vi "NGTS_DAQmx_Initialize_AI.vi"(7 "Save Virtual Channels":bool, 8 "error in":errorcluster, 10 "Channels Properties Table":string[][](array[string])) -> (0 "error out":errorcluster, 2 "AI Task Array Out":refnum<k21>[](array[refnum]))   [LabVIEW 2012]
doc: "Creates tasks based on \"Number_of_SCXI_Chassis\" entry in the AI_Configuration section of the Config_INI file. It then populates the tasks with Channels created from rows in the Channel Properties Table. The Tasks are optionally saved in MAX. If not, the the Auto Cleanup of Tasks is TRUE and LabVIEW will automatically clean up Tasks of completion of execution of the application.\n\n2007-11 Mike Ashe\nmichael.ashe@imaginatics.net\nCell: 860-961-0876"
panel:
  in  "Author":string="Mike Ashe"
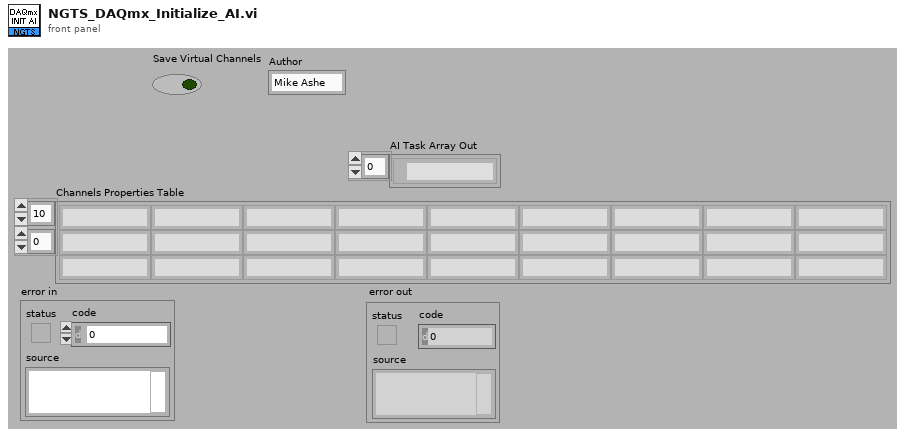
[diagram p1: front panel]
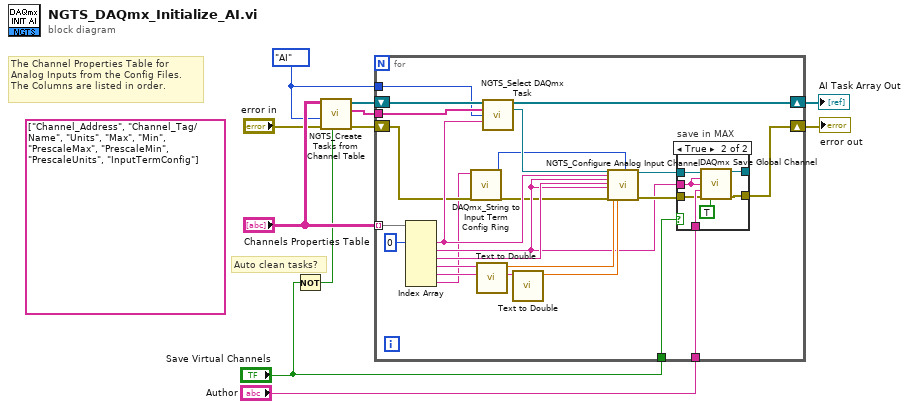
[diagram p0: block diagram]
diagram:
  w2 = enum16{"AI", "AO", "DI", "DO"}."AI" ("Type of IO")
  (unwired) string[] ["Channel_Address", "Channel_Tag/Name", "Units", "Max", "Min", "PrescaleMax", "PrescaleMin", "PrescaleUnits", "InputTermConfig"]
  # "Auto clean tasks?"
  # "The Channel Properties Table for\nAnalog Inputs from the Config Files.\nThe Columns are listed in order."
  n1 = Not(x="Save Virtual Channels") -> (.not. x?=w6:bool)
  n2 = call "NGTS_Create Tasks from Channel Table.vi"("Task Auto Cleanup?"=w6, "error in"="error in", "Type of IO"=w2, "Channels Properties Table"="Channels Properties Table") -> ("error out"=w4:errorcluster, "List of Devices"=w3:string[], "DAQmx Task Array Out"=w5:refnum<k21>[])  [unwired: 5 in]
  n3 = for {
    shift-right: [w17] -> w10
    shift-left: w5 -> [w21]
    tunnel: "Author" -> [w32]
    tunnel: "Save Virtual Channels" -> [w31]
    tunnel: "Channels Properties Table" -> [w30] mode=indexing
    shift-right: [w23] -> w9
    shift-left: w4 -> [w15]
    tunnel: w3 -> [w20]
    tunnel: w2 -> [w16]
    n4 = Index Array(array=w30, index #1=0 ("index")) -> (element #1=w19:string, element #2=w22:string, element #3=w29:string, element #4=w28:string, element #5=w27:string, element #6=w13:string)  [unwired: 5 in]
    n5 = call "DAQmx_String to Input Term Config Ring.vi"("error in (no error)"=w15, "Input TermCfg Str"=w13) -> ("error out"=w14:errorcluster, "input terminal configuration"=w12:i32)  [unwired: 8 in]
    n6 = call "Text to Double.vi"("string"=w28) -> ("number"=w26:dbl)  [unwired: 10 in]
    n7 = call "NGTS_Select DAQmx Task.vi"("DAQmx Tasks In"=w21, "List of Devices"=w20, "Type of IO"=w16, "Channel Address"=w19) -> ("DAQmx Tasks Out"=w17:refnum<k21>[], "DAQmx Task Selected Out"=w18:refnum<k21>)  [unwired: 9 in, 1 out]
    n8 = call "Text to Double.vi"("string"=w27) -> ("number"=w25:dbl)  [unwired: 10 in]
    n9 = call "NGTS_Configure Analog Input Channel.vi"("task in"=w18, "Channel Address"=w19, "Channel Name"=w22, "Units"=w29, "Custom Scale Name"=w22, "error in (no error)"=w14, "maximum value"=w26, "minimum value"=w25, "input terminal configuration"=w12) -> ("task out"=w33:refnum<k21>, "error out"=w34:errorcluster)  [unwired: 17 in]
    n10 = case "save in MAX" shown="True" w31 {
      tunnel: [w36 w43] -> _
      tunnel: w22 -> [_ w40]
      tunnel: w32 -> [_ w42]
      tunnel: [w35 w41] -> w23
      tunnel: w33 -> [w36 w39]
      tunnel: w34 -> [w35 w38]
      frame False {
      }
      frame True {
        n11 = call <vilib>:"DAQmx Save Global Channel.vi"("task/channels in"=w39, "channel name"=w40, "save as"=w40, "author"=w42, "error in"=w38, "overwrite existing channel?"=TRUE) -> ("task out"=w43:refnum<k21>, "error out"=w41:errorcluster)  [unwired: 8 in]
      }
    }
  }
  "AI Task Array Out" <- w10
  "error out" <- w9
